vi "DistGlobal.vi"() -> ()   [LabVIEW 2014]
panel:
  out "Distance":dbl
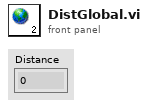
[diagram p1: front panel]
diagram:
